vi "IT6900 Output DC Volts.vi"() -> ()   [LabVIEW 2013]
uses:
  IT6900.lvlib
panel:
  in  "Serial Configuration":T1={"Baud Rate"=9600, "Parity"=0, "Data Bits"=8, "Stop Bits"=10, "Flow Control"=0} {"Flow Control" items=["None", "XON/XOFF", "RTS/CTS", "XON/XOFF & RTS/CTS", "DTR/DSR", "XON/XOFF & DTR/DSR"]; "Stop Bits" items=["1.0"=10, "1.5"=15, "2.0"=20]; "Data Bits" items=["7"=7, "8"=8]; "Parity" items=["None", "Odd", "Even", "Mark", "Space"]; "Baud Rate" items=["300"=300, "600"=600, "1200"=1200, "2400"=2400, "4800"=4800, "9600"=9600, "19200"=19200]}
  in  "Stop Output":bool
  in  "Voltage Level (0V)":dbl format="%.2f"
  out "Actual Current Level (A)":dbl format="%.3f"
  out "Actual Voltage Level (V)":dbl format="%.3f"
  in  "Current Level (0A)":dbl format="%.2f"
  in  "VISA resource name":refnum<visa-resource-name>
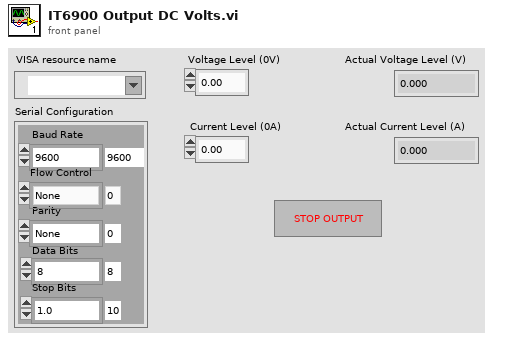
[diagram p1: front panel]
types:
  T1 = cluster{"Baud Rate":u32, "Parity":u16, "Data Bits":u16, "Stop Bits":u16, "Flow Control":u16}
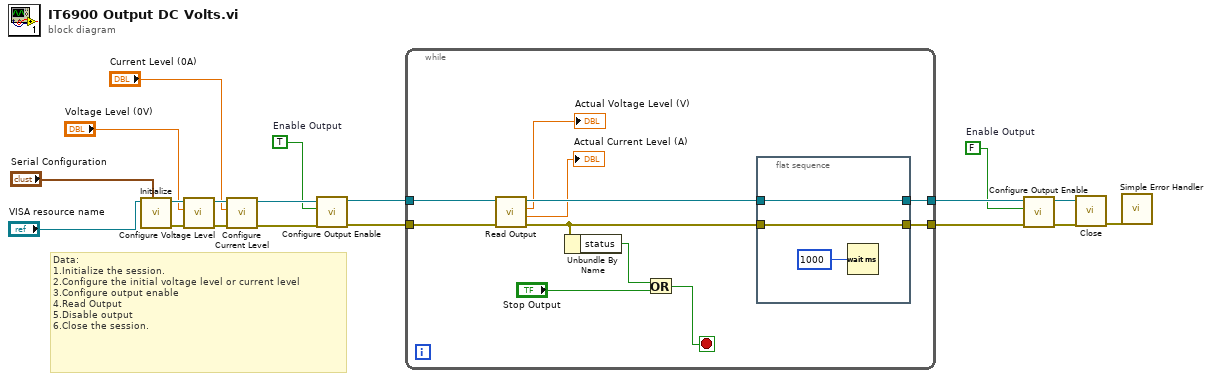
[diagram p0: block diagram]
diagram:
  w4 = FALSE  # Enable Output
  w5 = TRUE  # Enable Output
  # "Data:\n1.Initialize the session.\n2.Configure the initial voltage level or current level\n3.Configure output enable\n4.Read Output\n5.Disable output\n6.Close the session."
  n1 = call "Initialize.vi"("Serial Configuration"="Serial Configuration", "VISA resource name"="VISA resource name") -> ("error out"=w17:errorcluster, "VISA resource name out"=w16:refnum<visa-resource-name>)  [unwired: 8 in]
  n2 = call "Configure Voltage Level.vi"("error in (no error)"=w17, "Voltage Level (0.0 V)"="Voltage Level (0V)", "VISA resource name"=w16) -> ("error out"=w14:errorcluster, "VISA resource name out"=w13:refnum<visa-resource-name>)  [unwired: 7 in]
  n3 = call "Configure Current Level.vi"("error in (no error)"=w14, "Current Level (0.0 A)"="Current Level (0A)", "VISA resource name"=w13) -> ("error out"=w10:errorcluster, "VISA resource name out"=w11:refnum<visa-resource-name>)  [unwired: 7 in]
  n4 = call "Configure Output Enable.vi"("VISA resource name"=w11, "Enable Output (T: Enable)"=w5, "error in (no error)"=w10) -> ("VISA resource name out"=w9:refnum<visa-resource-name>, "error out"=w8:errorcluster)  [unwired: 6 in]
  n5 = while {
    tunnel: w9 -> [w25]
    tunnel: w8 -> [w24]
    tunnel: [w27] -> w7
    tunnel: [w26] -> w6
    stop <- w28 stop-if-true
    n6 = call "Read Output.vi"("error in (no error)"=w24, "VISA resource name"=w25) -> ("error out"=w22:errorcluster, "Actual Current Level (0.0A)"=→"Actual Current Level (A)":dbl, "Actual Voltage Level (0.0V)"=→"Actual Voltage Level (V)":dbl, "VISA resource name out"=w23:refnum<visa-resource-name>)  [unwired: 6 in]
    n7 = Unbundle By Name(w22) -> ("status"=w30:bool)
    n8 = Or(x=w30, y="Stop Output") -> (x .or. y?=w28:bool)
    n9 = flat-sequence {
      tunnel: w23 -> [w32]
      tunnel: [w32] -> w27
      tunnel: [w31] -> w26
      tunnel: w22 -> [w31]
      frame #0 {
        n10 = Wait (ms)(milliseconds to wait=1000) -> ()  [unwired: 1 out]
      }
    }
  }
  n11 = call "Configure Output Enable.vi"("VISA resource name"=w7, "Enable Output (T: Enable)"=w4, "error in (no error)"=w6) -> ("VISA resource name out"=w2:refnum<visa-resource-name>, "error out"=w3:errorcluster)  [unwired: 6 in]
  n12 = call "Close.vi"("error in (no error)"=w3, "VISA resource name"=w2) -> ("error out"=w1:errorcluster)  [unwired: 9 in]
  n13 = call <vilib>:"Simple Error Handler.vi"("error in (no error)"=w1) -> ()  [unwired: 4 in, 5 out]
